vi "Raise Packet Timeout Error.vi"(8 "error in (no error)":errorcluster, 10 "Enable Packet Timeout Error":bool, 11 "VISA resource name":refnum<visa-resource-name>) -> (0 "error out":errorcluster, 3 "VISA resource name out":refnum<visa-resource-name>)   [LabVIEW 2020, in "ZaberTSeries.lvlib"]
doc: "Set the error state for a partial packet timeout. Does nothing if <b>Enable Packet Timeout Error</b> is false."
uses:
  ZaberTSeries.lvlib
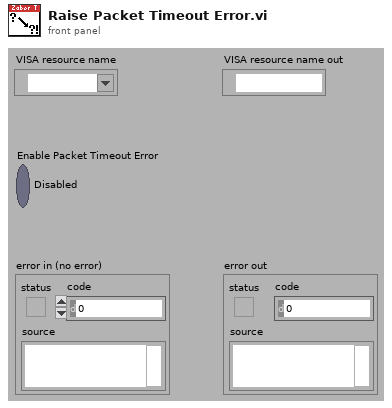
[diagram p1: front panel]
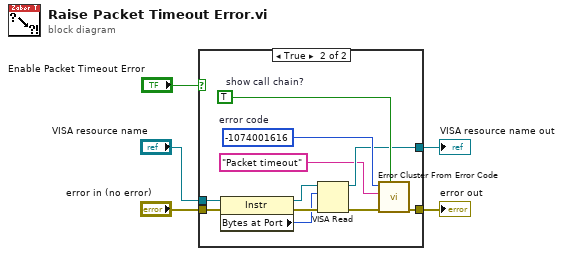
[diagram p0: block diagram]
diagram:
  n1 = case shown="True" "Enable Packet Timeout Error" {
    tunnel: "error in (no error)" -> [w7 w11]
    tunnel: [w7 w14] -> w3
    tunnel: "VISA resource name" -> [w6 w13]
    tunnel: [w6 w16] -> w5
    frame False {
    }
    frame True {
      w17 = -1074001616  # error code
      w18 = TRUE  # show call chain?
      n2 = property class="Instr"(reference=w13, error in=w11) -> (reference out=w12:refnum<visa-resource-name>, error out=w10:errorcluster, "Bytes at Port"=w9:u32)
      n3 = VISA Read(VISA resource name=w12, byte count=w9, error in (no error)=w10) -> (VISA resource name out=w16:refnum<visa-resource-name>, error out=w15:errorcluster)  [unwired: 2 out]
      n4 = call "Error Cluster From Error Code.vi"("show call chain? (False)"=w18, "error in (no error)"=w15, "error message (\"\")"="Packet timeout" ("error message (\"\")"), "error code (0)"=w17) -> ("error out"=w14:errorcluster)  [unwired: 5 in]
    }
  }
  "VISA resource name out" <- w5
  "error out" <- w3
